vi "Move from S.vi"(10 "Position in":cluster{i32, i32}, 11 "Map in":T1(c390)) -> (2 "Position out":cluster{i32, i32}, 3 "Map out":T1(c390))   [LabVIEW 2023, in "d10.lvlib"]
uses:
  d10.lvlib
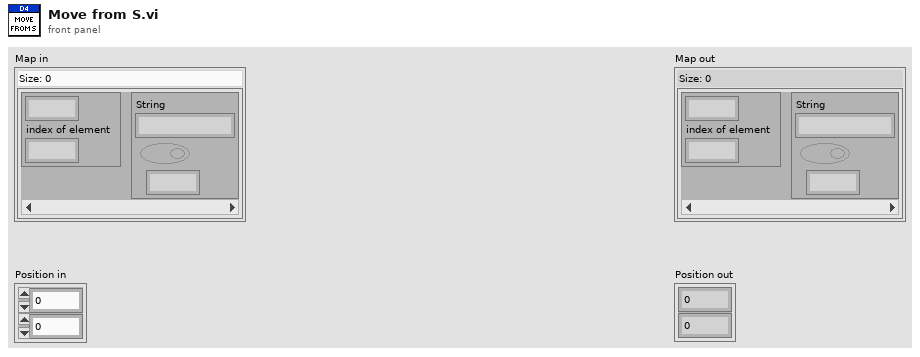
[diagram p1: front panel]
types:
  T1 = map{cluster{i32, "index of element":i32}, cluster{"String":string, bool, u64}}
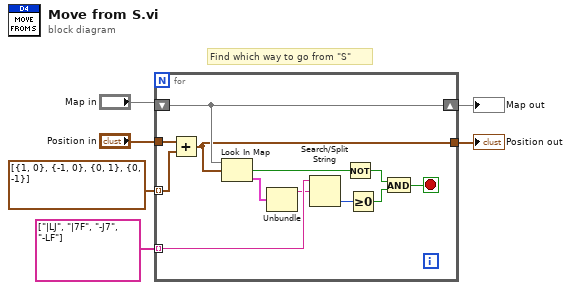
[diagram p0: block diagram]
diagram:
  # "Find which way to go from \"S\""
  n1 = for {
    tunnel: cluster{i32, i32}[] [{1, 0}, {-1, 0}, {0, 1}, {0, -1}] -> [w17] mode=indexing
    tunnel: "Position in" -> [w18]
    tunnel: string[] ["|LJ", "|7F", "-J7", "-LF"] -> [w16] mode=indexing
    shift-right: [w15] -> w6
    shift-left: "Map in" -> [w15]
    tunnel: [w8] -> w3
    stop <- w7 stop-if-true
    n2 = Add(x=w18, y=w17) -> (x+y=w8:cluster{i32, i32})
    n3 = Look In Map(map=w15, key=w8) -> (key not found?=w14:bool, value=w13:cluster{"String":string, bool, u64})  [unwired: 1 in]
    n4 = Unbundle(w13) -> ("String"=w12:string)  [unwired: 2 out]
    n5 = Search/Split String(string=w16, search string/char (-)=w12) -> (offset of match=w11:i32)  [unwired: 1 in, 2 out]
    n6 = Not(x=w14) -> (.not. x?=w10:bool)
    n7 = Greater Or Equal To 0?(x=w11) -> (x >= 0?=w9:bool)
    n8 = And(x=w10, y=w9) -> (x .and. y?=w7:bool)
  }
  "Position out" <- w3
  "Map out" <- w6
